vi "pessimize_objective_fun_cno.vi"(9 "output selector":T1, 10 "data":T2, 11 "X":dbl[](array[numeric])) -> (0 "error out":errorcluster, 1 "inequality constraint function values":dbl[](array[numeric]), 2 "equality constraint function values":dbl[](array[numeric]), 3 "objective function value":dbl)   [LabVIEW 2013]
doc: "This template is the starting point for creating an objective function, equality constraint function and inequality constraint function to be passed to the Constrained Nonlinear Optimization.vi."
uses:
  <vilib>/gmath/NumericalOptimization/objective function data.ctl
  <vilib>/gmath/NumericalOptimization/cno_output select.ctl
  <vilib>/gmath/NI_Gmath.lvlib
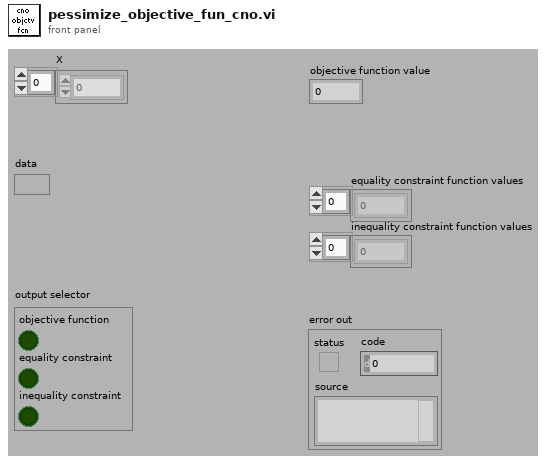
[diagram p1: front panel]
types:
  T1 = typedef "NI_Gmath.lvlib/cno_output select.ctl" = cluster{"objective function":bool, "equality constraint":bool, "inequality constraint":bool}
  T2 = typedef "NI_Gmath.lvlib/objective function data.ctl" = variant
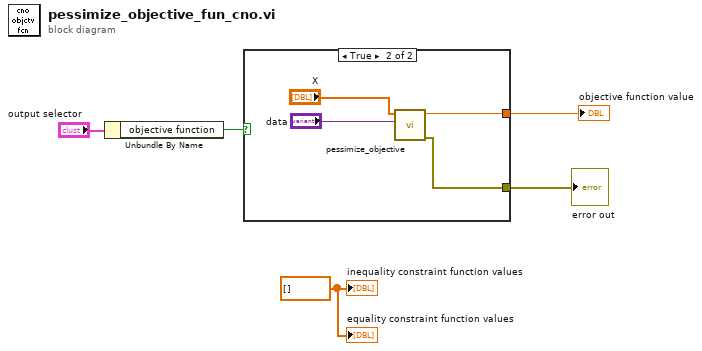
[diagram p0: block diagram]
diagram:
  w2 = dbl[] [] ("inequality constraint function values")
  n1 = Unbundle By Name("output selector") -> ("objective function"=w1:bool)
  n2 = case shown="True" w1 {
    tunnel: [_ w8] -> w4
    tunnel: [_ w7] -> w3
    frame False {
    }
    frame True {
      n3 = call "pessimize_objective.vi"("data"="data", "X"="X") -> ("error out"=w7:errorcluster, "f(X)"=w8:dbl)  [unwired: 7 in, 1 out]
    }
  }
  "objective function value" <- w4
  "error out" <- w3
  "equality constraint function values" <- w2
  "inequality constraint function values" <- w2
